vi "newEndValue.vi"(8 "error in (no error)":errorcluster, 11 "RampAction in":refnum<class "RampAction.lvclass">) -> (0 "error out":errorcluster, 3 "RampAction out":refnum<class "RampAction.lvclass">)   [LabVIEW 2011, in "Views.lvlib" / "ScriptEditor.lvlib" / "RampAction.lvclass"]
uses:
  RampAction.lvclass
  RampAction.lvclass/RampAction.ctl
  Tools/Scripting/ScriptingEvent/ScriptEvent.lvclass
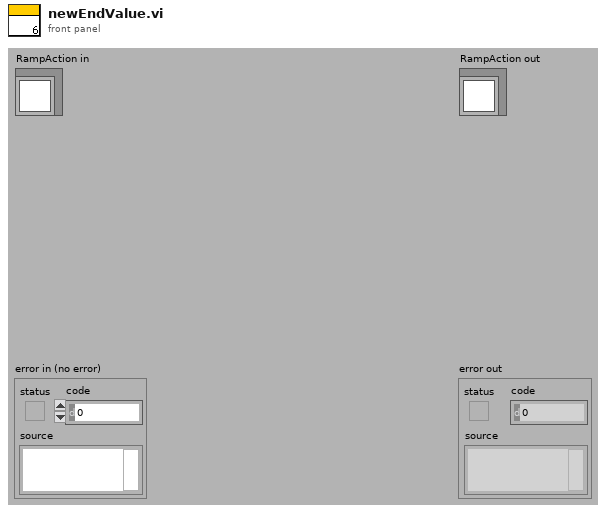
[diagram p1: front panel]
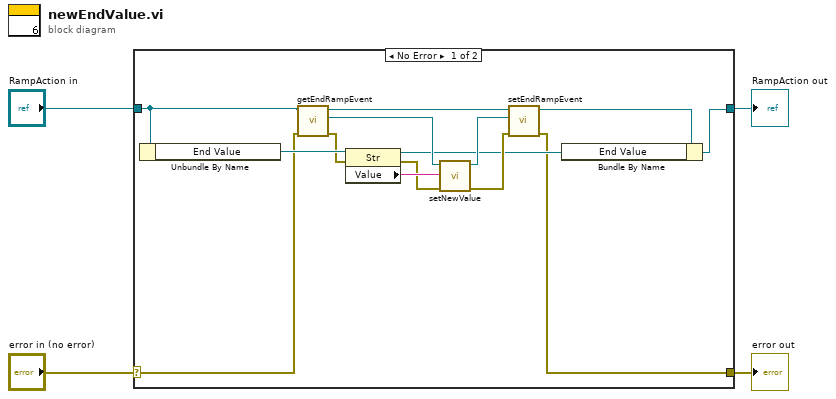
[diagram p0: block diagram]
diagram:
  n1 = case shown="No Error" "error in (no error)" {
    selector: "error in (no error)" -> [w6 w20]
    tunnel: [w5 w20] -> w3
    tunnel: [w7 w19] -> w1
    tunnel: "RampAction in" -> [w18 w19]
    frame No Error {
      n2 = Unbundle By Name(w18) -> ("End Value"=w17:refnum<vi>)
      n3 = call "getEndRampEvent.vi"("error in (no error)"=w6, "RampAction in"=w18) -> ("error out"=w16:errorcluster, "EndScriptEvent"=w15:refnum<class "ScriptEvent.lvclass">, "RampAction out"=w12:refnum<class "RampAction.lvclass">)  [unwired: 7 in]
      n4 = property class="Str"(reference=w17, error in=w16) -> (reference out=w9:refnum<vi>, error out=w13:errorcluster, "Value"=w14:string)
      n5 = call "setNewValue.vi"("error in (no error)"=w13, "newValue"=w14, "ScriptEvent.lvclass in"=w15) -> ("error out"=w11:errorcluster, "ScriptEvent.lvclass out"=w10:refnum<class "ScriptEvent.lvclass">)  [unwired: 7 in]
      n6 = call "setEndRampEvent.vi"("error in (no error)"=w11, "EndScriptEvent"=w10, "RampAction in"=w12) -> ("error out"=w5:errorcluster, "RampAction out"=w8:refnum<class "RampAction.lvclass">)  [unwired: 7 in]
      n7 = Bundle By Name(cluster=w8, "End Value"=w9) -> (w7:refnum<class "RampAction.lvclass">)
    }
    frame Error {
    }
  }
  "error out" <- w3
  "RampAction out" <- w1
